vi "PitchSlider.vi"(4 "Y Resolution":i32, 5 "Min":dbl, 6 "X Resolution":i32, 7 "Max":dbl, 8 "Load":dbl, 9 "Shoot":dbl, 10 "Current":dbl, 11 "Image In":T1) -> (3 "Image Out":T1)   [LabVIEW 2012]
uses:
  <vilib>/vision/Image Controls.llb/IMAQ Image.ctl
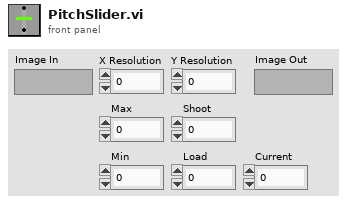
[diagram p1: front panel]
types:
  T1 = typedef "IMAQ Image.ctl" = refnum<image>
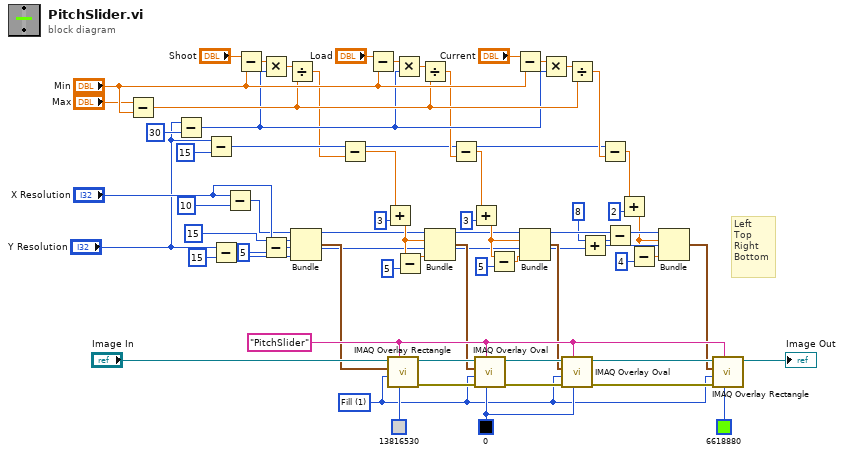
[diagram p0: block diagram]
diagram:
  w31 = 8 ("y")
  w46 = u32 0 ("Color")
  w48 = "PitchSlider"
  w45 = u32 1 items=["Frame", "Fill", "Highlight"] ("Drawing Mode (Frame)")
  # "Left\nTop\nRight\nBottom"
  n1 = Subtract(x="Max", y="Min") -> (x-y=w12:dbl)
  n2 = Subtract(x="Y Resolution", y=30) -> (x-y=w10:i32)
  n3 = Subtract(x="Y Resolution", y=15) -> (x-y=w3:i32)
  n4 = Subtract(x="Y Resolution", y=15) -> (x-y=w59:i32)
  n5 = Subtract(x="X Resolution", y=10) -> (x-y=w32:i32)
  n6 = Subtract(x="Shoot", y="Min") -> (x-y=w18:dbl)
  n7 = Multiply(x=w18, y=w10) -> (x*y=w21:dbl)
  n8 = Subtract(x="X Resolution", y=5) -> (x-y=w30:i32)
  n9 = Divide(x=w21, y=w12) -> (x/y=w2:dbl)
  n10 = Bundle(w32, 15, w30, w59) -> (w41:cluster{i32, i32, i32, i32})  [unwired: 1 in]
  n11 = Subtract(x=w3, y=w2) -> (x-y=w1:dbl)
  n12 = Subtract(x="Load", y="Min") -> (x-y=w16:dbl)
  n13 = Add(x=w1, y=3) -> (x+y=w36:dbl)
  n14 = call "IMAQ Overlay Rectangle"("Color"=u32 13816530, "Group"=w48, "Drawing Mode (Frame)"=w45, "Rectangle"=w41, "Image"="Image In") -> ("error out"=w51:errorcluster, "Image Out"=w55:T1)  [unwired: 5 in]
  n15 = Multiply(x=w16, y=w10) -> (x*y=w20:dbl)
  n16 = Subtract(x=w36, y=5) -> (x-y=w39:dbl)
  n17 = Divide(x=w20, y=w12) -> (x/y=w7:dbl)
  n18 = Bundle(w32, w36, w30, w39) -> (w43:cluster{i32, dbl, i32, dbl})  [unwired: 1 in]
  n19 = Subtract(x=w3, y=w7) -> (x-y=w6:dbl)
  n20 = Add(x=w6, y=3) -> (x+y=w33:dbl)
  n21 = call "IMAQ Overlay Oval"("Color"=w46, "Group"=w48, "error in (no error)"=w51, "Drawing Mode (Frame)"=w45, "Bounding Rectangle"=w43, "Image"=w55) -> ("error out"=w50:errorcluster, "Image Out"=w54:T1)  [unwired: 4 in]
  n22 = Subtract(x=w33, y=5) -> (x-y=w37:dbl)
  n23 = Subtract(x="Current", y="Min") -> (x-y=w15:dbl)
  n24 = Bundle(w32, w33, w30, w37) -> (w42:cluster{i32, dbl, i32, dbl})  [unwired: 1 in]
  n25 = Multiply(x=w15, y=w10) -> (x*y=w19:dbl)
  n26 = call "IMAQ Overlay Oval"("Color"=w46, "Group"=w48, "error in (no error)"=w50, "Drawing Mode (Frame)"=w45, "Bounding Rectangle"=w42, "Image"=w54) -> ("error out"=w49:errorcluster, "Image Out"=w53:T1)  [unwired: 4 in]
  n27 = Divide(x=w19, y=w12) -> (x/y=w4:dbl)
  n28 = Add(x=w31, y=w30) -> (x+y=w28:i32)
  n29 = Subtract(x=w3, y=w4) -> (x-y=w5:dbl)
  n30 = Subtract(x=w32, y=w31) -> (x-y=w29:i32)
  n31 = Add(x=w5, y=2) -> (x+y=w24:dbl)
  n32 = Subtract(x=w24, y=4) -> (x-y=w26:dbl)
  n33 = Bundle(w29, w24, w28, w26) -> (w23:cluster{i32, dbl, i32, dbl})  [unwired: 1 in]
  n34 = call "IMAQ Overlay Rectangle"("Color"=u32 6618880, "Group"=w48, "error in (no error)"=w49, "Drawing Mode (Frame)"=w45, "Rectangle"=w23, "Image"=w53) -> ("Image Out"=→"Image Out":T1)  [unwired: 4 in, 1 out]
